vi "pierwszy program VI.vi"() -> ()   [LabVIEW 2020]
panel:
  out "sum":dbl
  in  "numeric array":dbl[][][][][][](array[numeric])
  out "y 3":dbl
  out "y 2":dbl
  in  "x":dbl
  in  "y":dbl
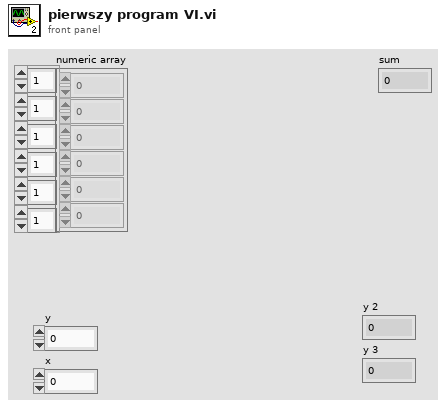
[diagram p1: front panel]
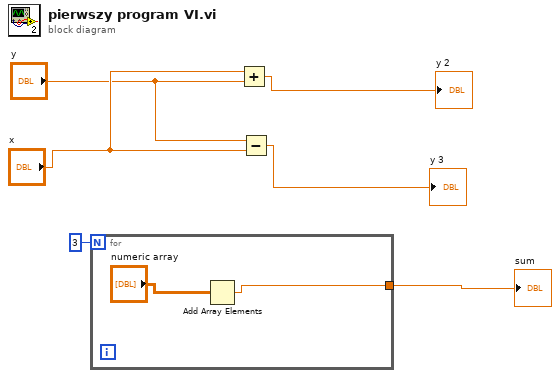
[diagram p0: block diagram]
diagram:
  n1 = for {
    N: 3 -> [_]
    tunnel: [w8] -> w2
    n2 = Add Array Elements(numeric array="numeric array") -> (sum=w8:dbl)
  }
  "sum" <- w2
  n3 = Add(x="x", y="y") -> (x+y=→"y 2":dbl)
  n4 = Subtract(x="y", y="x") -> (x-y=→"y 3":dbl)
